vi "Pcre2GetMatchOffsetsOfSubstringNumber8.vi"(8 "error in":errorcluster, 9 "Number":i32, 10 "MatchResult":i32=-1, 11 "pMatchData":u64 format="%.0x") -> (0 "error out":errorcluster, 1 "OffsetPastMatch":i32, 2 "MatchOffset":i32, 3 "pMatchData":u64 format="%.0x")   [LabVIEW 2021, in "libpcre2-8.lvlib"]
uses:
  libpcre2-8.lvlib
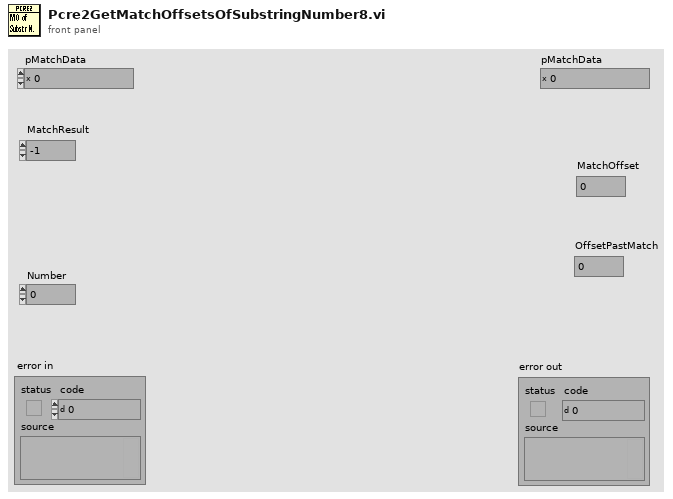
[diagram p1: front panel]
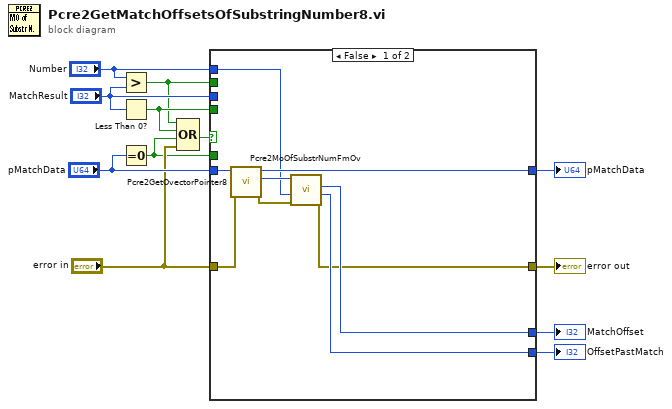
[diagram p0: block diagram]
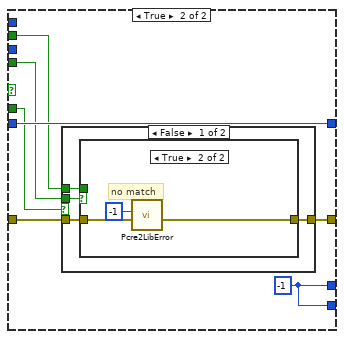
[diagram p2: hidden frame]
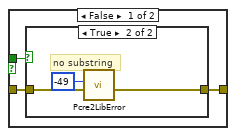
[diagram p3: hidden frame]
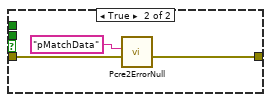
[diagram p5: hidden frame]
diagram:
  n1 = Greater?(x="Number", y="MatchResult") -> (0:w1:bool)
  n2 = Less Than 0?(x="MatchResult") -> (x < 0?=w5:bool)
  n3 = Equal To 0?(x="pMatchData") -> (x = 0?=w4:bool)
  n4 = Compound Arithmetic op=OR(w1, w5, w4, "error in") -> (w7:bool)
  n5 = case shown="False" w7 {
    tunnel: "error in" -> [w19 w25]
    tunnel: [w13 w27] -> w12
    tunnel: "pMatchData" -> [w21 w28]
    tunnel: [w20 w28] -> w11
    tunnel: [w14 w22] -> w9
    tunnel: [w15 w22] -> w8
    tunnel: "MatchResult" -> [_ _]
    tunnel: w5 -> [_ w24]
    tunnel: w4 -> [_ w26]
    tunnel: "Number" -> [w16 _]
    tunnel: w1 -> [_ w23]
    frame False {
      n6 = call "Pcre2GetOvectorPointer8.vi"("error in"=w19, "pMatchData"=w21) -> ("error out"=w17:errorcluster, "pOvector"=w18:u64, "pMatchData"=w20:u64)  [unwired: 7 in]
      n7 = call "Pcre2MoOfSubstrNumFmOv.vi"("error in"=w17, "Number"=w16, "pOvector"=w18) -> ("error out"=w13:errorcluster, "OffsetPastMatch"=w15:i32, "MatchOffset"=w14:i32)  [unwired: 5 in, 1 out]
    }
    frame True {
      w22 = -1
      n8 = case shown="False" w26 {
        tunnel: w25 -> [w31 w44]
        tunnel: [w30 w43] -> w27
        tunnel: w24 -> [w32 _]
        tunnel: w23 -> [w29 _]
        frame False {
          n9 = case shown="True" w32 {
            tunnel: w31 -> [w34 w42]
            tunnel: [w33 w41] -> w30
            tunnel: w29 -> [w35 _]
            frame False {
              n10 = case shown="True" w35 {
                tunnel: w34 -> [w36 w38]
                tunnel: [w36 w39] -> w33
                frame False {
                }
                frame True {
                  # "no substring"
                  n11 = call "Pcre2LibError.vi"("error in"=w38, "ErrorCode"=-49) -> ("error out"=w39:errorcluster)  [unwired: 9 in]
                }
              }
            }
            frame True {
              # "no match"
              n12 = call "Pcre2LibError.vi"("error in"=w42, "ErrorCode"=-1) -> ("error out"=w41:errorcluster)  [unwired: 9 in]
            }
          }
        }
        frame True {
          n13 = call "Pcre2ErrorNull.vi"("error in"=w44, "What"="pMatchData") -> ("error out"=w43:errorcluster)  [unwired: 9 in]
        }
      }
    }
  }
  "pMatchData" <- w11
  "error out" <- w12
  "MatchOffset" <- w9
  "OffsetPastMatch" <- w8
